vi "acquisition loop.vi"(8 "error in":errorcluster, 9 "notifier data":refnum<notifier>, 10 "Data Queue":refnum<queue>, 11 "Message Queues":T1) -> (0 "error out":errorcluster)   [LabVIEW 2017, in "Acquisition.lvlib"]
uses:
  Acquisition.lvlib
  Control/Message Queues.ctl
  flow_control_3.0.0/flow_queue_datatype.ctl
  Control/Config chanel.ctl
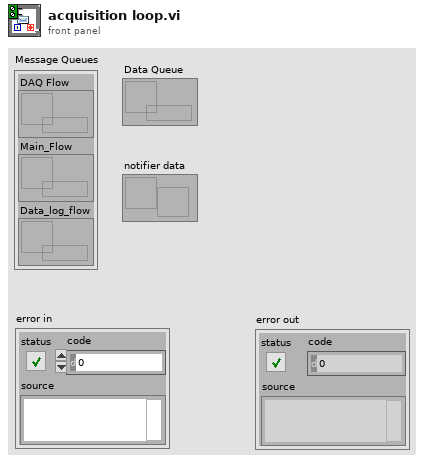
[diagram p1: front panel]
types:
  T1 = typedef "Message Queues.ctl" = cluster{"DAQ Flow":refnum<queue>, "Main_Flow":refnum<queue>, "Data_log_flow":refnum<queue>}
  T2 = typedef "Config chanel.ctl" = cluster{"Hardware config":cluster{"DAQmx Channel":tag, "Minimum Input":dbl, "Maximum Input":dbl, "Sampling Rate":dbl, "Samples Read":dbl, "DAQmx Task Name":refnum<k21>}, "Path":path}
  T3 = typedef "flow_queue_datatype.ctl" = cluster{"command":string, "parameter":variant}
  T4 = cluster{"DAQmx Channel":tag, "Minimum Input":dbl, "Maximum Input":dbl, "Sampling Rate":dbl, "Samples Read":dbl, "DAQmx Task Name":refnum<k21>}
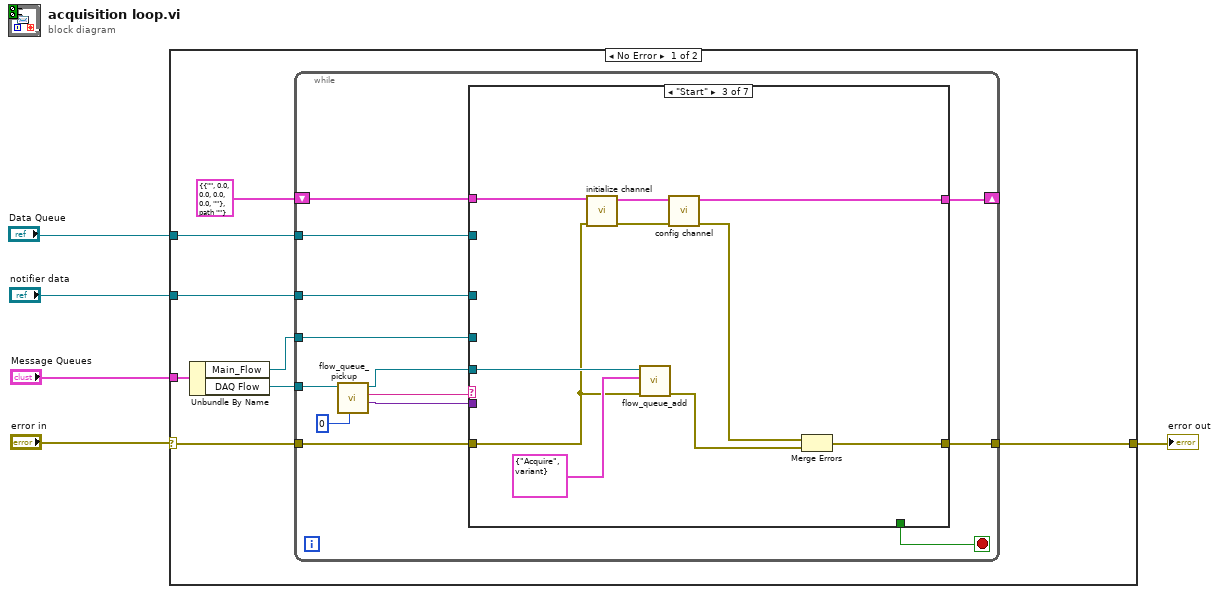
[diagram p0: block diagram]
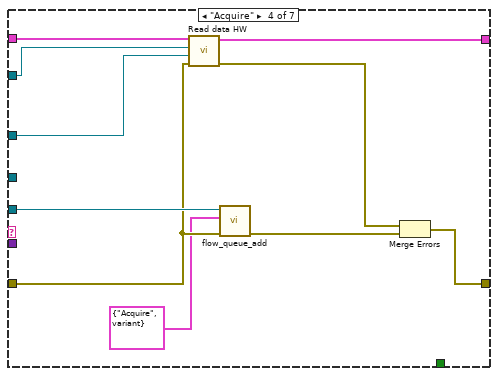
[diagram p4: hidden frame]
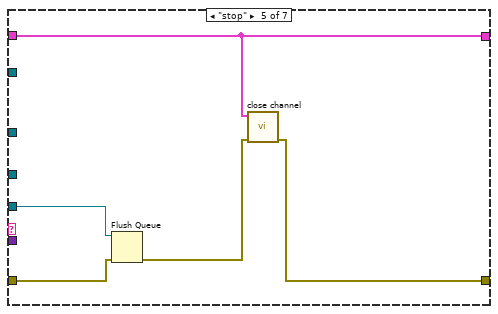
[diagram p5: hidden frame]
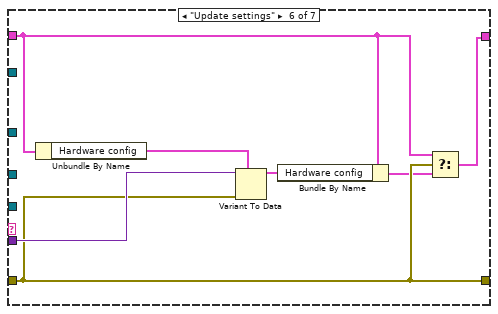
[diagram p6: hidden frame]
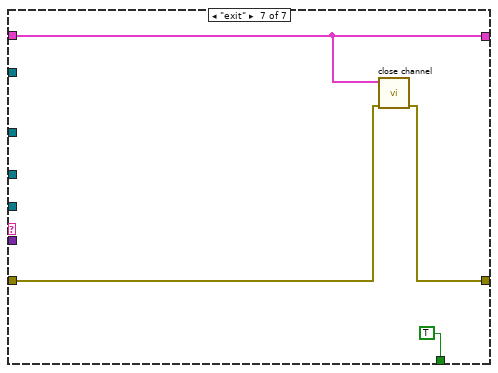
[diagram p7: hidden frame]
diagram:
  n1 = case shown="No Error" "error in" {
    selector: "error in" -> [w11 w67]
    tunnel: "Message Queues" -> [w13 _]
    tunnel: [w6 w67] -> w3
    tunnel: "Data Queue" -> [w9 _]
    tunnel: "notifier data" -> [w8 _]
    frame No Error {
      n2 = Unbundle By Name(w13) -> ("Main_Flow"=w10:refnum<queue>, "DAQ Flow"=w12:refnum<queue>)
      n3 = while {
        tunnel: w12 -> [w26]
        tunnel: w11 -> [w24]
        shift-right: [w21] -> _
        shift-left: T2 {"Hardware config"={"DAQmx Channel"="", "Minimum Input"=0.0, "Maximum Input"=0.0, "Sampling Rate"=0.0, "Samples Read"=0.0, "DAQmx Task Name"=""}, "Path"=path ""} ("DAQ config") -> [w22]
        tunnel: [w20] -> w6
        tunnel: w10 -> [w18]
        tunnel: w9 -> [w16]
        tunnel: w8 -> [w15]
        stop <- w17 stop-if-true
        n4 = call "flow_queue_pickup.vi"("timeout"=0, "queue in"=w26) -> ("parameter"=w19:variant, "command"=w25:string, "queue out"=w23:refnum<queue>)  [unwired: 5 in, 2 out]
        n5 = case shown="\"Start\"" w25 {
          tunnel: w24 -> [w27 w29 w35 w45 w52 w61 w64]
          tunnel: w23 -> [_ _ w37 w46 w55 _ _]
          tunnel: w22 -> [w28 w30 w40 w50 w54 w56 w65]
          tunnel: [w28 w30 w31 w49 w54 w60 w65] -> w21
          tunnel: [w27 w29 w32 w47 w51 w61 w63] -> w20
          tunnel: w19 -> [_ _ _ _ _ w62 _]
          tunnel: w18 -> [_ _ _ _ _ _ _]
          tunnel: [_ _ _ _ _ _ TRUE] -> w17
          tunnel: w16 -> [_ _ _ w42 _ _ _]
          tunnel: w15 -> [_ _ _ w41 _ _ _]
          frame Default {
          }
          frame "Initialize" {
          }
          frame "Start" {
            n6 = call "initialize channel.vi"("error in"=w35, "DAQ Config"=w40) -> ("error out"=w38:errorcluster, "DAQ Config out"=w39:T2)  [unwired: 8 in]
            n7 = call "flow_queue_add.vi"("error in"=w35, "data"=T3 {"command"="Acquire", "parameter"=variant}, "queue in"=w37) -> ("error out"=w33:errorcluster)  [unwired: 7 in, 1 out]
            n8 = call "config channel.vi"("error in"=w38, "DAQ Config"=w39) -> ("error out"=w34:errorcluster, "DAQ Config out"=w31:T2)  [unwired: 8 in]
            n9 = Merge Errors(w34, w33) -> (w32:errorcluster)
          }
          frame "Acquire" {
            n10 = call "Read data HW.vi"("error in"=w45, "notifier data"=w41, "Data Queue"=w42, "HW Resource in"=w50) -> ("error out"=w48:errorcluster, "HW Resource out"=w49:T2)  [unwired: 6 in]
            n11 = call "flow_queue_add.vi"("error in"=w45, "data"=T3 {"command"="Acquire", "parameter"=variant}, "queue in"=w46) -> ("error out"=w43:errorcluster)  [unwired: 7 in, 1 out]
            n12 = Merge Errors(w48, w43) -> (w47:errorcluster)
          }
          frame "stop" {
            n13 = Flush Queue(queue=w55, error in (no error)=w52) -> (error out=w53:errorcluster)  [unwired: 2 out]
            n14 = call "close channel.vi"("error in"=w53, "DAQ Config"=w54) -> ("error out"=w51:errorcluster)  [unwired: 9 in]
          }
          frame "Update settings" {
            n15 = Unbundle By Name(w56) -> ("Hardware config"=w59:T4)
            n16 = Variant To Data(error in=w61, type=w59, Variant=w62) -> (data=w58:T4)  [unwired: 1 out]
            n17 = Bundle By Name(cluster=w56, "Hardware config"=w58) -> (w57:T2)
            n18 = Select(t=w56, s=w61, f=w57) -> (s? t:f=w60:T2)
          }
          frame "exit" {
            n19 = call "close channel.vi"("error in"=w64, "DAQ Config"=w65) -> ("error out"=w63:errorcluster)  [unwired: 9 in]
          }
        }
      }
    }
    frame Error {
    }
  }
  "error out" <- w3
